vi "Find Text.vi"(10 "Caller Reference":refnum<vi>, 11 "String Reference":refnum<vi>) -> ()   [LabVIEW 2014]
doc: "This VI displays a dialog allowing the user to search a text display for a specified string.\nA reference to the string control must be passed in.\nWhen the string is found, the calling VI will become front-most so the string can be highlighted.\nIf the string is not found, an error message is displayed.\nSearching starts from the cursor location in the text control.\nYou can change the search direction using the radial buttons.\nThe VI will remember previous search strings inside the combo box where you enter the text to find.\nIf you pass in a caller reference, this will be used to center the dialog. Otherwise, the VI will attempt to find it's caller in the call chain and center on that. If you call this VI dynamically, it will center itself on the primary monitor if the caller reference is not passed in."
uses:
  <vilib>/Utility/miscctls.llb/LVComboBoxStrsAndValuesArrayTypeDef.ctl
panel:
  in  "Direction":enum32{"reverse", "forward"}(radio)=enum."forward"
  in  "case sensitive?":bool
  in  "Find":bool
  in  "Find what:":string(combo)
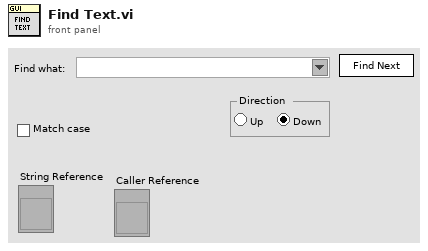
[diagram p1: front panel]
types:
  T1 = typedef "LVComboBoxStrsAndValuesArrayTypeDef.ctl" = cluster{"String":string, "Value":string}[]
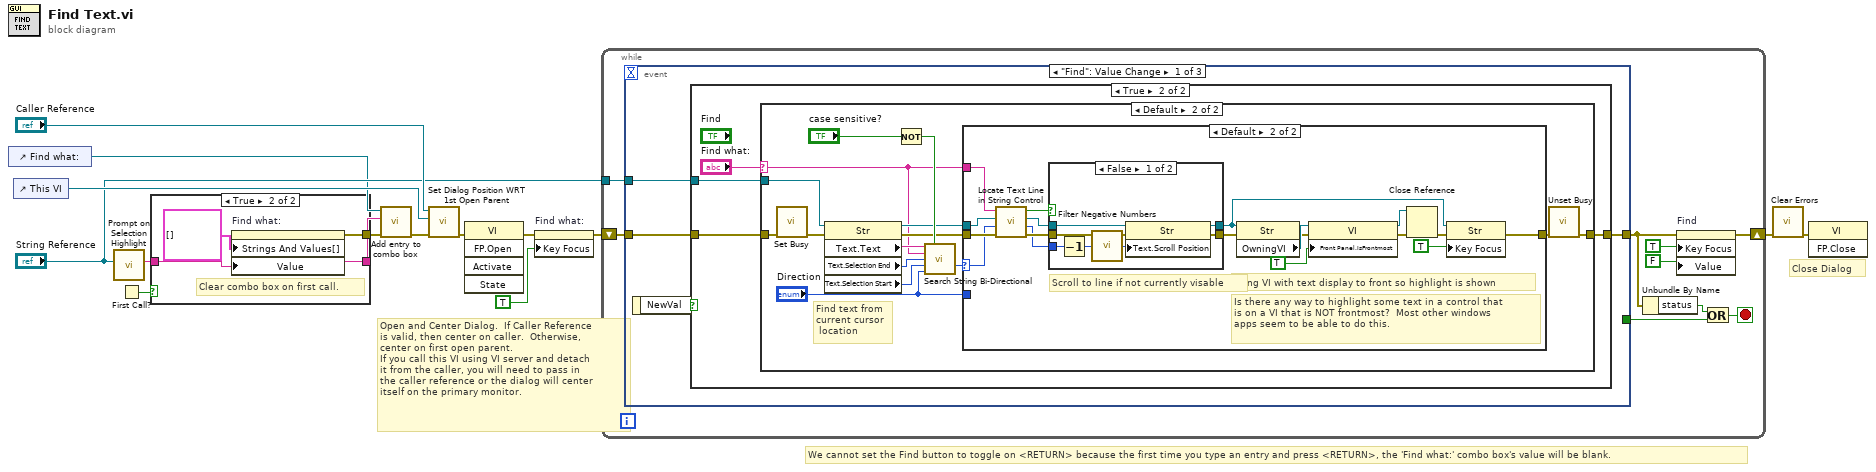
[diagram p0: block diagram]
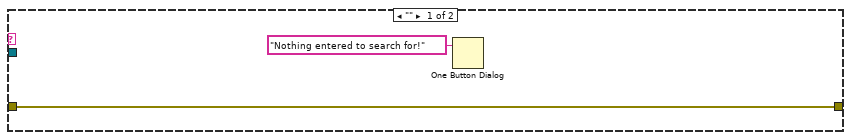
[diagram p4: hidden frame]
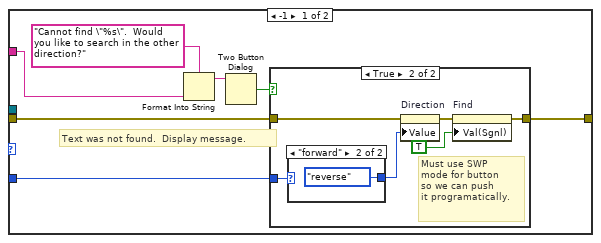
[diagram p5: hidden frame]
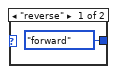
[diagram p7: hidden frame]
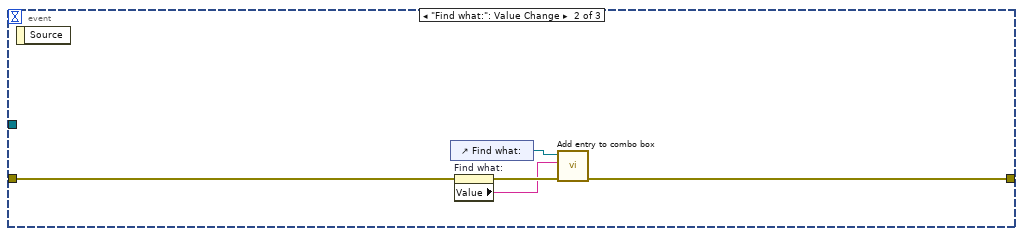
[diagram p9: hidden frame]
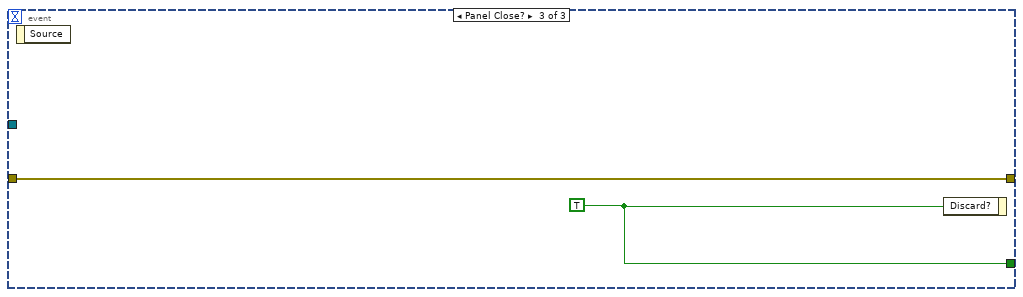
[diagram p10: hidden frame]
diagram:
  # "We cannot set the Find button to toggle on <RETURN> because the first time you type an entry and press <RETURN>, the 'Find what:' combo box's value will be blank."
  # "Close Dialog"
  # "Open and Center Dialog.  If Caller Reference\nis valid, then center on caller.  Otherwise,\ncenter on first open parent.\nIf you call this VI using VI server and detach\nit from the caller, you will need to pass in\nthe caller reference or the dialog will center\nitself on the primary monitor."
  n1 = control-ref of="Find what:"() -> (w1:refnum<vi>)
  n2 = control-ref of="This VI"() -> (w15:refnum<vi>)
  n3 = call "Prompt on Selection Highlight.vi"("String Reference In"="String Reference") -> ("Starting String"=w5:string)  [unwired: 6 out]
  n4 = First Call?() -> (First Call?: T/F=w9:bool)
  n5 = case shown="True" w9 {
    tunnel: [_ w19] -> w3
    tunnel: w5 -> [w16 w17]
    tunnel: [w16 w17] -> w2
    frame False {
    }
    frame True {
      # "Clear combo box on first call."
      n6 = property on="Find what:" class="CmbBox"("Strings And Values[]"=T1 [] ("Strings And Values []"), "Value"=w17) -> (error out=w19:errorcluster)  [unwired: 2 in, 1 out]
    }
  }
  n7 = call "Add entry to combo box.vi"("error in"=w3, "Value"=w2, "CmbBox Refnum"=w1) -> ("error out"=w4:errorcluster)  [unwired: 4 out]
  n8 = call "Set Dialog Position WRT 1st Open Parent.vi"("error in"=w4, "Dialog Reference"=w15, "Caller Reference"="Caller Reference") -> ("error out"=w10:errorcluster)  [unwired: 4 out]
  n9 = invoke class="VI" method="FP.Open"(error in=w10) -> (error out=w8:errorcluster)  [unwired: 4 in, 4 out]
  n10 = property on="Find what:" class="CmbBox"(error in=w8, "Key Focus"=TRUE) -> (error out=w11:errorcluster)  [unwired: 1 in, 1 out]
  n11 = while {
    shift-right: [w24] -> w14
    shift-left: w11 -> [w27]
    tunnel: "String Reference" -> [w20]
    stop <- w26 stop-if-true
    n12 = event shown="[0] \"Find\": Value Change" {
      selector: _ -> [_ _ _]
      dyn-events: _ -> [_ _ _]
      timeout: _ -> [_ _ _]
      tunnel: [_ _ w104] -> w28
      tunnel: w27 -> [w32 w101 w103]
      tunnel: [w31 w102 w103] -> w23
      tunnel: w20 -> [w29 _ _]
      event "Find": Value Change {
        n13 = event-data() -> ("NewVal"=w30:bool)  [unwired: 1 out]
        n14 = case shown="True" w30 {
          tunnel: w32 -> [w33 w37]
          tunnel: [w33 w36] -> w31
          tunnel: w29 -> [_ w35]
          frame False {
            # "Find not TRUE.  Ignore Value Change event."
          }
          frame True {
            n15 = case shown="Default" "Find what:" {
              selector: "Find what:" -> [_ w40]
              tunnel: w37 -> [w39 w54]
              tunnel: [w39 w42] -> w36
              tunnel: w35 -> [_ w41]
              frame "" {
                n16 = One Button Dialog(message="Nothing entered to search for!" ("format string")) -> ()  [unwired: 2 out]
              }
              frame Default {
                # "Find text from\ncurrent cursor\n location"
                n17 = call <vilib>:"Set Busy.vi"("error in (no error)"=w54) -> ("error out"=w43:errorcluster)  [unwired: 3 in, 7 out]
                n18 = property class="Str"(reference=w41, error in=w43) -> (reference out=w45:refnum<vi>, error out=w46:errorcluster, "Text.Text"=w47:string, "Text.Selection End"=w51:u32, "Text.Selection Start"=w50:u32)
                n19 = Not(x="case sensitive?") -> (.not. x?=w52:bool)
                n20 = call "Search String Bi-Directional.vi"("Input String"=w47, "Ignore Case?"=w52, "Search String"=w40, "Selection End"=w51, "Selection Start"=w50, "Direction"="Direction") -> ("Offset in String"=w49:i32)  [unwired: 9 out]
                n21 = case shown="Default" w49 {
                  selector: w49 -> [_ w84]
                  tunnel: w45 -> [_ w85]
                  tunnel: w46 -> [w57 w88]
                  tunnel: [w55 w87] -> w44
                  tunnel: w40 -> [w59 w86]
                  tunnel: "Direction" -> [w58 _]
                  frame -1 {
                    # "Text was not found.  Display message."
                    n22 = Format Into String(format string="Cannot find \"%s\".  Would you like to search in the other direction?", w59) -> (resulting string=w60:string)  [unwired: 2 in, 1 out]
                    n23 = Two Button Dialog(message=w60) -> (T button?=w56:bool)  [unwired: 2 out]
                    n24 = case shown="True" w56 {
                      tunnel: w58 -> [_ w68]
                      tunnel: w57 -> [w62 w64]
                      tunnel: [w62 w63] -> w55
                      frame False {
                      }
                      frame True {
                        # "Must use SWP\nmode for button\nso we can push\nit programatically."
                        n25 = case shown="\"forward\"" w68 {
                          tunnel: [enum32{"reverse", "forward"}."forward" ("Direction") enum32{"reverse", "forward"}."reverse" ("Direction")] -> w67
                          frame "reverse" {
                          }
                          frame "forward" {
                          }
                        }
                        n26 = property on="Direction" class="RadioBtnsControl (strict)"(error in=w64, "Value"=w67) -> (error out=w66:errorcluster)  [unwired: 1 in, 1 out]
                        n27 = property on="Find" class="Bool (strict)"(error in=w66, "Val(Sgnl)"=TRUE) -> (error out=w63:errorcluster)  [unwired: 1 in, 1 out]
                      }
                    }
                  }
                  frame Default {
                    # "Is there any way to highlight some text in a control that\nis on a VI that is NOT frontmost?  Most other windows\napps seem to be able to do this."
                    # "Bring VI with text display to front so highlight is shown"
                    # "Scroll to line if not currently visable"
                    n28 = call "Locate Text Line in String Control.vi"("error in"=w88, "Offset in String"=w84, "String Reference In"=w85, "Find what:"=w86) -> ("error out"=w83:errorcluster, "Scroll Position"=w80:i32, "String Reference Out"=w82:refnum<vi>, "In View?"=w81:bool)  [unwired: 2 in, 2 out]
                    n29 = case shown="False" w81 {
                      tunnel: w80 -> [w95 _]
                      tunnel: w83 -> [w94 w97]
                      tunnel: w82 -> [w93 w96]
                      tunnel: [w92 w96] -> w78
                      tunnel: [w91 w97] -> w77
                      frame False {
                        n30 = Decrement(x=w95) -> (x-1=w90:i32)
                        n31 = call "Filter Negative Numbers.vi"("Numeric In"=w90) -> ("Numeric Out"=w89:i32)  [unwired: 4 out]
                        n32 = property class="Str"(reference=w93, error in=w94, "Text.Scroll Position"=w89) -> (reference out=w92:refnum<vi>, error out=w91:errorcluster)
                      }
                      frame True {
                      }
                    }
                    n33 = property class="Str"(reference=w78, error in=w77) -> (error out=w75:errorcluster, "OwningVI"=w76:refnum<vi>)  [unwired: 1 out]
                    n34 = property class="VI"(reference=w76, error in=w75, "Front Panel.IsFrontmost"=TRUE ("Front Panel Window:Is Frontmost")) -> (reference out=w72:refnum<vi>, error out=w73:errorcluster)
                    n35 = Close Reference(reference=w72, error in (no error)=w73) -> (error out=w71:errorcluster)
                    n36 = property class="Str"(reference=w78, error in=w71, "Key Focus"=TRUE) -> (error out=w87:errorcluster)  [unwired: 1 out]
                  }
                }
                n37 = call <vilib>:"Unset Busy.vi"("error in (no error)"=w44) -> ("error out"=w42:errorcluster)  [unwired: 1 in, 9 out]
              }
            }
          }
        }
      }
      event "Find what:": Value Change {
        n38 = event-data() -> ()  [unwired: 2 out]
        n39 = control-ref of="Find what:"() -> (w98:refnum<vi>)
        n40 = property on="Find what:" class="CmbBox"(error in=w101) -> (error out=w100:errorcluster, "Value"=w99:string)  [unwired: 1 in, 1 out]
        n41 = call "Add entry to combo box.vi"("error in"=w100, "Value"=w99, "CmbBox Refnum"=w98) -> ("error out"=w102:errorcluster)  [unwired: 4 out]
      }
      event Panel Close? {
        w104 = TRUE ("Discard?")
        n42 = event-data() -> ()  [unwired: 2 out]
        n43 = event-data("Discard?"=w104) -> ()  [unwired: 1 in, 1 out]
      }
    }
    n44 = Unbundle By Name(w23) -> ("status"=w25:bool)
    n45 = property on="Find" class="Bool (strict)"(error in=w23, "Key Focus"=TRUE, "Value"=FALSE ("Key Focus")) -> (error out=w24:errorcluster)  [unwired: 1 in, 1 out]
    n46 = Or(x=w25, y=w28) -> (x .or. y?=w26:bool)
  }
  n47 = call <vilib>:"Clear Errors.vi"("error in (no error)"=w14) -> ("error out"=w13:errorcluster)  [unwired: 1 in, 5 out]
  n48 = invoke class="VI" method="FP.Close"(error in=w13) -> ()  [unwired: 2 in, 3 out]
